vi "Baud Rate Detect.vi"() -> ()   [LabVIEW 2011]
doc: "ID=0x6009"
uses:
  VIs/g_data.ctl
  data/ControlCAN.dll
panel:
  out "label2 4":string="CAN中继状态"
  out "label2 3":string="CAN中继状态"
  out "label2 2":string="CAN中继状态"
  out "label2":string="CAN中继状态"
  in  "help":bool
  in  "close":bool
  in  "DevInd":u32(ring) caption="Device index:" items=["0", "1", "2", "3", "4"]
  in  "SAM":u8(ring) caption="Sample:" items=["Sampling 1 time", "Sampling 3 times"]
  in  "SJW":u8(ring)=1 caption="SJW:" items=["1TQ"=1, "2TQ"=2, "3TQ"=3, "4TQ"=4]
  in  "detect_n":bool
  in  "g_e":dbl=1000.0 caption="To" min=10.0 max=1000.0 step=0.001
  in  "g_b":dbl=10.0 caption="From" min=10.0 max=1000.0 step=0.001
  in  "VCI_CAN_STATUS":T1
  out "Success":bool
  in  "stop":bool
  in  "apply":bool
  in  "detect":bool
  in  "list":i32(listbox)
  in  "Run":bool
  in  "Channel":u32(ring) caption="Channel:" items=["Ch1", "Ch2"]
  in  "DevType":u32(ring)=3 caption="Device type:" items=["USB-CAN"=3, "USB-CAN 2.0"=4]
  # "Kbps"
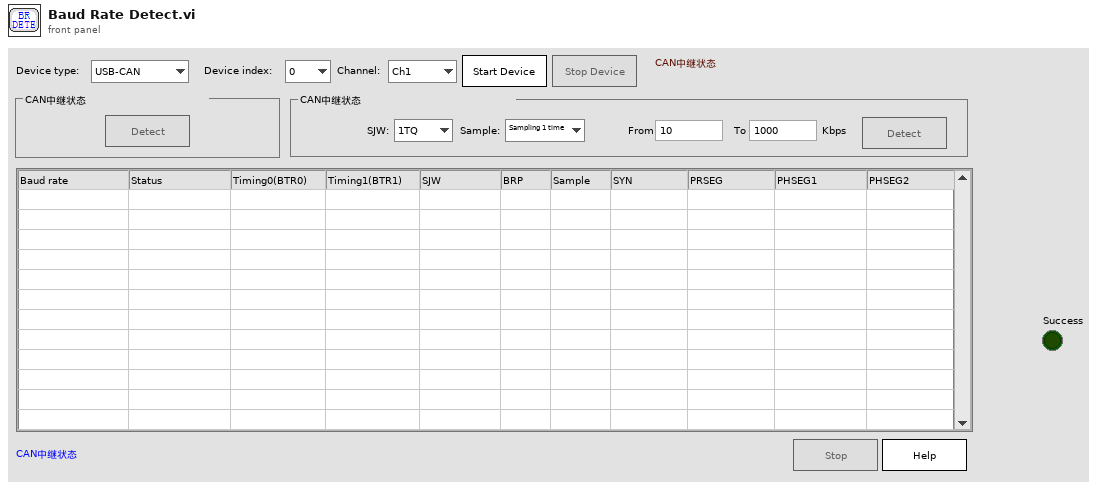
[diagram p1: front panel]
types:
  T1 = cluster{"ErrInterrupt":u8, "regMode":u8, "regStatus":u8, "regALCapture":u8, "regECCapture":u8, "regEWLimit":u8, "regRECounter":u8, "regTECounter":u8, "Reserved":u32}
  T2 = typedef "Baud rate Self Define.ctl" = cluster{"BAUD":u32, "SJW":u8, "BRP":u8, "SAM":u8, "PHS2_SEL":u8, "SYN(nouse)":u8, "PRSEG":u8, "PHSEG1":u8, "PHSEG2":u8}
  T3 = cluster{"AccCode":u32, "AccMask":u32, "Reserved":u32, "Filter":u8, "Timing0":u8, "Timing1":u8, "Mode":u8}
  T4 = typedef "g_data.ctl" = cluster{"b":dbl, "e":dbl}
  T5 = enum8{"Enabled", "Disabled", "Disabled and Grayed Out"}
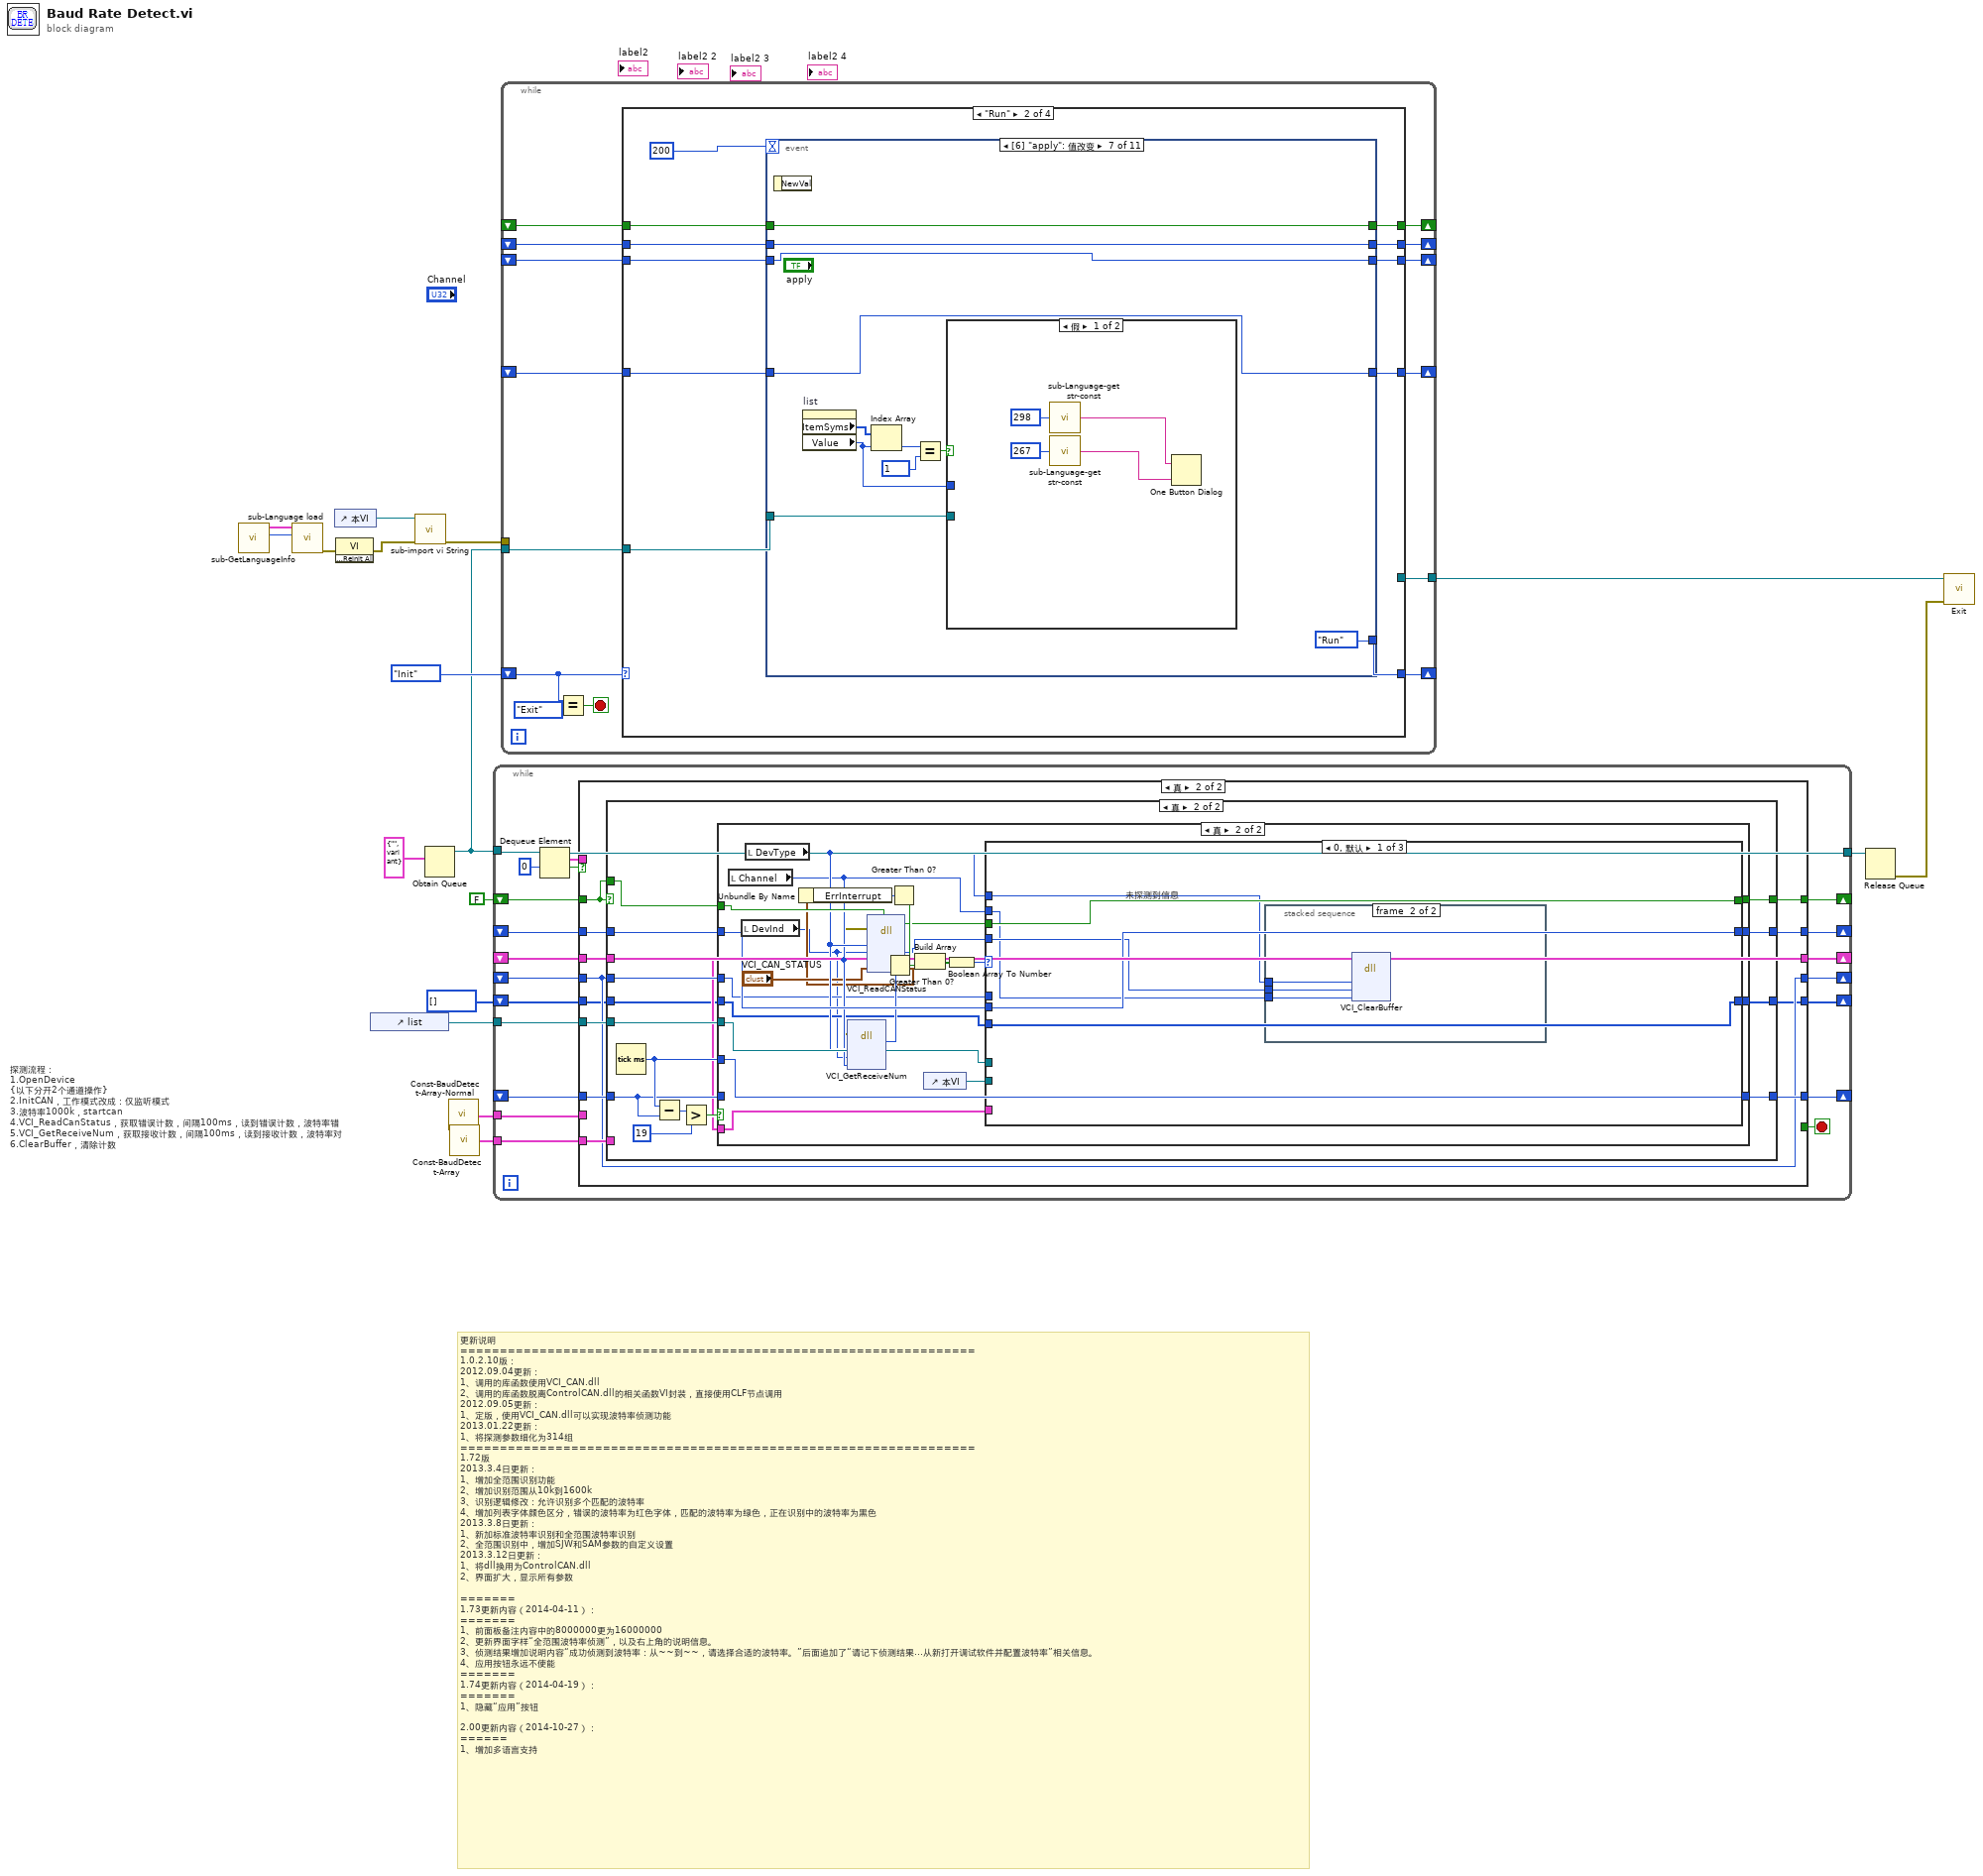
[diagram p0: block diagram]
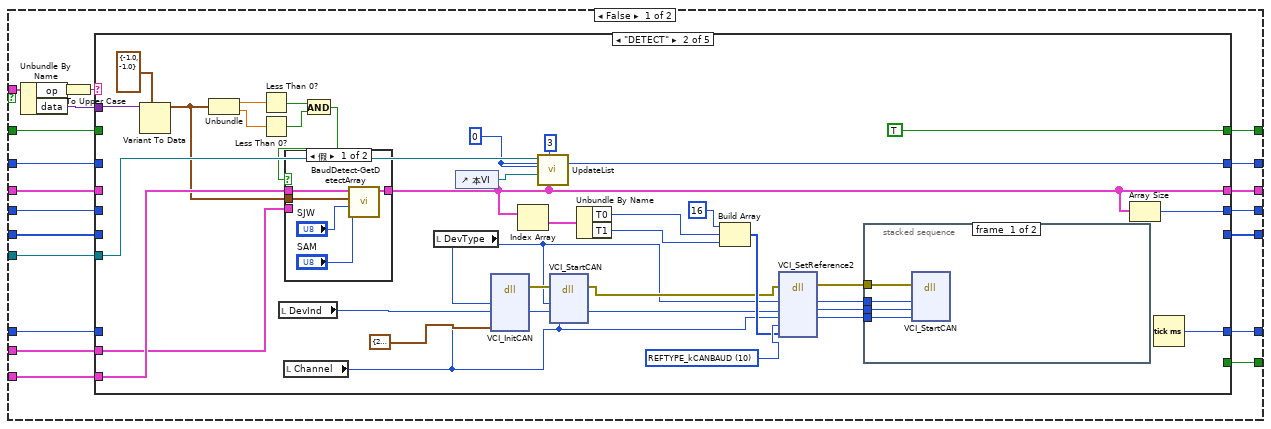
[diagram p2: hidden frame]
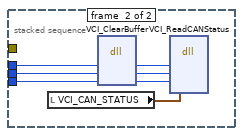
[diagram p4: hidden frame]
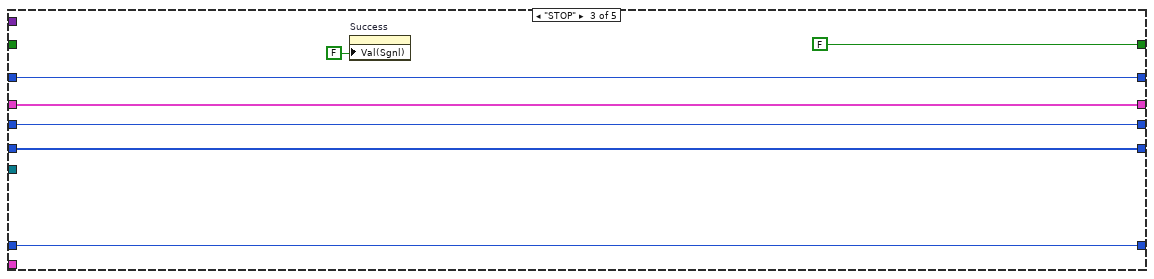
[diagram p6: hidden frame]
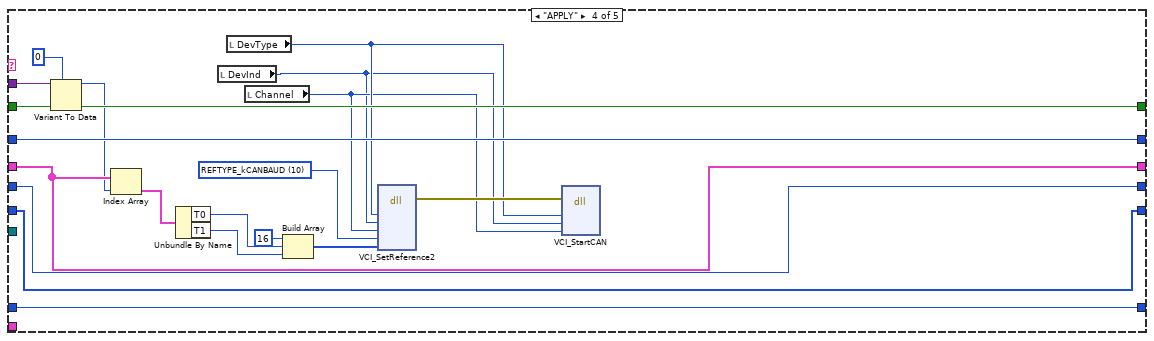
[diagram p7: hidden frame]
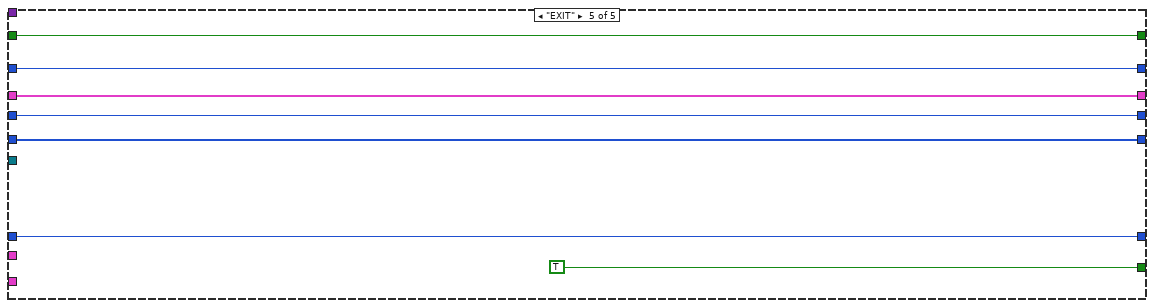
[diagram p8: hidden frame]
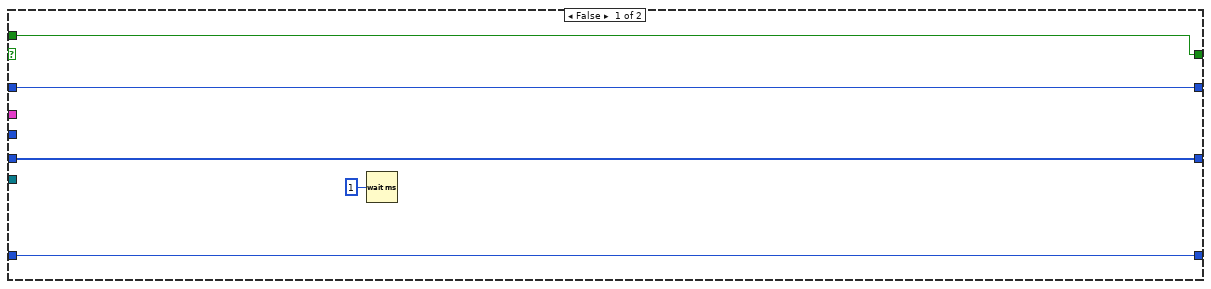
[diagram p9: hidden frame]
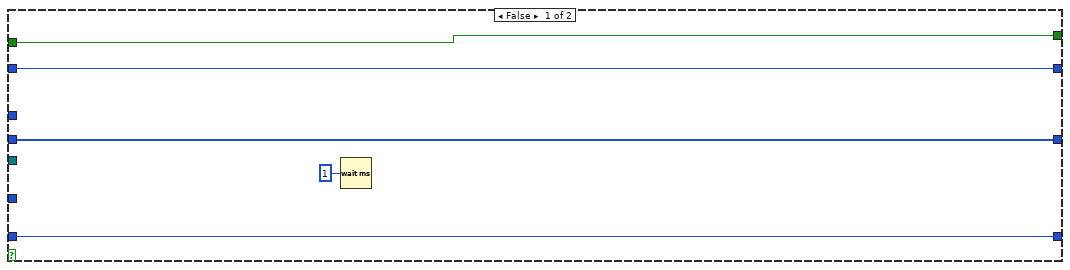
[diagram p10: hidden frame]
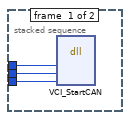
[diagram p11: hidden frame]
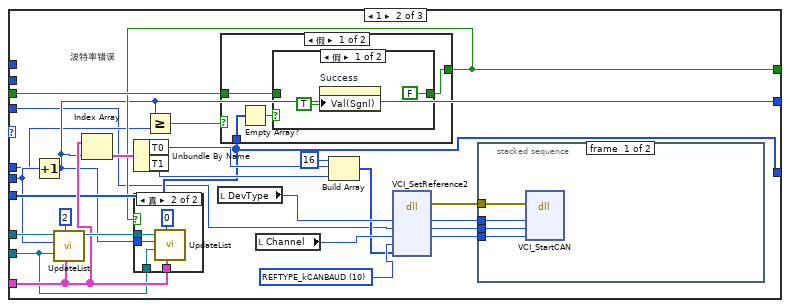
[diagram p12: hidden frame]
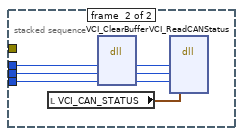
[diagram p14: hidden frame]
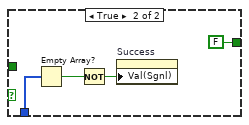
[diagram p16: hidden frame]
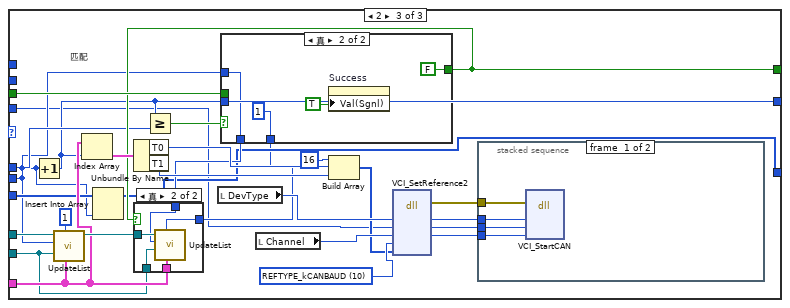
[diagram p17: hidden frame]
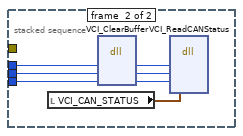
[diagram p19: hidden frame]
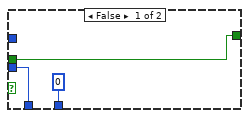
[diagram p20: hidden frame]
diagram:
  # "更新说明\n=================================================================\n1.0.2.10版：\n2012.09.04更新：\n1、调用的库函数使用VCI_CAN.dll\n2、调用的库函数脱离ControlCAN.dll的相关函数VI封装，直接使用CLF节点调用\n2012.09.05更新：\n1、定版，使用VCI_CAN.dll可以实现波特率侦测功能\n2013.01.22更新：\n1、将探测参数细化为314组\n=================================================================\n1.72版\n2013.3.4日更新：\n1、增加全范围识别功能\n2、增加识别范围从10k到1600k\n3、识别逻辑修改：允许识别多个匹配的波特率\n4、增加列表字体颜色区分，错误的波特率为红色字体，匹配的波特率为绿色，正在识别中的波特率为黑色\n2013.3.8日更新：\n1、新加标准波特率识别和全范围波特率识别\n2、全范围识别中，增加SJW和SAM参数的自定义设置\n2013.3.12日更新：\n1、将dll换用为ControlCAN.dll\n2、界面扩大，显示所有参数\n\n=======\n1.73更新内容（2014-04-11）：\n=======\n1、前面板备注内容中的8000000更为16000000\n2、更新界面字样“全范围波特率侦测”，以及右上角的说明信息。\n3、侦测结果增加说明内容“成功侦测到波特率：从~~到~~，请选择合适的波特率。”后面追加了“请记下侦测结果...从新打开调试软件并配置波特率”相关信息。\n4、应用按钮永远不使能\n=======\n1.74更新内容（2014-04-19）：\n=======\n1、隐藏“应用”按钮\n\n2.00更新内容（2014-10-27）：\n======\n1、增加多语言支持"
  # "探测流程：\n1.OpenDevice\n{以下分开2个通道操作}\n2.InitCAN，工作模式改成：仅监听模式\n3.波特率1000k，startcan\n4.VCI_ReadCanStatus，获取错误计数，间隔100ms，读到错误计数，波特率错\n5.VCI_GetReceiveNum，获取接收计数，间隔100ms，读到接收计数，波特率对\n6.ClearBuffer，清除计数"
  n1 = call "sub-GetLanguageInfo.vi"() -> ("selected"=w1:i32, "languages"=w5:cluster{string, "appended path":path, string}[])  [unwired: 10 in]
  n2 = call "sub-Language load.vi"("selected"=w1, "languages"=w5) -> ("error out"=w2:errorcluster)  [unwired: 9 in]
  n3 = control-ref of="本VI"() -> (w6:refnum<vi>)
  n4 = invoke class="VI" method="Default Vals.Reinit All"(error in=w2) -> (error out=w3:errorcluster)  [unwired: 2 in, 2 out]
  n5 = control-ref of="list"() -> (w13:refnum<vi>)
  n6 = call "sub-import vi String.vi"("error in (no error)"=w3, "vi ref"=w6) -> ("error out"=w4:errorcluster)  [unwired: 9 in]
  n7 = Obtain Queue(element data type=cluster{"op":string, "data":variant} {"op"="", "data"=variant}) -> (queue out=w16:refnum<queue>)  [unwired: 4 in, 2 out]
  n8 = call "Const-BaudDetect-Array-Normal.vi"() -> ("DetectArray Nml"=w7:cluster{"T0":u8, "T1":u8, "br_selfdef":T2}[])
  n9 = call "Const-BaudDetect-Array.vi"() -> ("DetectArray"=w10:cluster{"T0":u8, "T1":u8, "br_selfdef":T2}[])
  n10 = while {
    tunnel: w16 -> [w34]
    tunnel: [w33] -> w15
    shift-right: [w31] -> _
    shift-left: FALSE -> [w32]
    shift-right: [w29] -> _
    shift-left: _ -> [w30]
    shift-right: [w28] -> _
    shift-left: _ -> [w27]
    tunnel: w13 -> [w26]
    tunnel: w10 -> [w25]
    shift-right: [w23] -> _
    shift-left: _ -> [w22]
    shift-right: [w21] -> _
    shift-left: _ -> [w24]
    shift-right: [w19] -> _
    shift-left: i32[] [] -> [w20]
    tunnel: w7 -> [w18]
    stop <- w35 stop-if-true
    n11 = Dequeue Element(queue=w34, timeout in ms (-1)=0 ("超时毫秒(-1)")) -> (queue out=w33:refnum<queue>, element=w36:cluster{"op":string, "data":variant}, timed out?=w37:bool)  [unwired: 1 in, 1 out]
    n12 = case shown="真" w37 {
      tunnel: w36 -> [w58 _]
      tunnel: [w56 _] -> w35
      tunnel: w32 -> [w55 w157]
      tunnel: [w54 w156] -> w31
      tunnel: w30 -> [w53 w160]
      tunnel: [w52 w159] -> w29
      tunnel: [w51 w161] -> w28
      tunnel: w27 -> [w50 w162]
      tunnel: w26 -> [w49 w158]
      tunnel: w25 -> [w48 w155]
      tunnel: w24 -> [w47 w153]
      tunnel: [w44 w154] -> w23
      tunnel: w22 -> [w43 w154]
      tunnel: [w42 w153] -> w21
      tunnel: w20 -> [w41 w152]
      tunnel: [w40 w151] -> w19
      tunnel: w18 -> [w39 _]
      frame False {
        n13 = Unbundle By Name(w58) -> ("op"=w46:string, "data"=w45:variant)
        n14 = To Upper Case(1:w46) -> (0:w57:string)
        n15 = case shown="\"DETECT\"" w57 {
          tunnel: [_ _ _ _ TRUE] -> w56
          tunnel: w55 -> [w64 _ _ w143 w149]
          tunnel: [w64 TRUE FALSE w143 w149] -> w54
          tunnel: w53 -> [w63 _ w124 w141 w148]
          tunnel: [w63 w95 w124 w141 w148] -> w52
          tunnel: [w62 w99 w123 w142 w147] -> w51
          tunnel: w50 -> [w62 _ w123 w142 w147]
          tunnel: w49 -> [_ w98 _ _ _]
          tunnel: w48 -> [_ w92 _ _ _]
          tunnel: w47 -> [w60 _ w119 w135 w145]
          tunnel: w45 -> [_ w94 _ w133 _]
          tunnel: [w61 w74 w120 w131 w146] -> w44
          tunnel: w43 -> [w61 _ w120 w131 w146]
          tunnel: [w60 w91 w119 w135 w145] -> w42
          tunnel: w41 -> [w59 _ w118 w134 w144]
          tunnel: [w59 _ w118 w134 w144] -> w40
          tunnel: w39 -> [_ w83 _ _ _]
          frame "假", Default {
          }
          frame "DETECT" {
            w82 = u32 10 items=["REFTYPE_MODE"=0, "REFTYPE_FILTER"=1, "REFTYPE_ACR0"=2, "REFTYPE_AMR0"=6, "REFTYPE_kCANBAUD"=10, "REFTYPE_CANRX_EN"=13, "REFTYPE_UARTBAUD"=14, "REFTYPE_ALL"=15] ("RefType")
            w95 = 0 ("t")
            n16 = Variant To Data(type=T4 {"b"=-1.0, "e"=-1.0} ("g_data"), Variant=w94) -> (data=w89:T4)  [unwired: 1 in, 1 out]
            n17 = Unbundle(w89) -> ("b"=w88:dbl, "e"=w87:dbl)
            n18 = Less Than 0?(x=w88) -> (x < 0?=w86:bool)
            n19 = Less Than 0?(x=w87) -> (x < 0?=w85:bool)
            n20 = local read "DevInd"() -> (w66:u32)
            n21 = local read "Channel"() -> (w65:u32)
            n22 = And(x=w86, y=w85) -> (x .and. y?=w84:bool)
            n23 = case shown="假" w84 {
              tunnel: w92 -> [w116 _]
              tunnel: [w115 w117] -> w74
              tunnel: w89 -> [w114 _]
              tunnel: w83 -> [_ w117]
              frame False {
                n24 = call "BaudDetect-GetDetectArray.vi"("SAM"="SAM", "SJW"="SJW", "g_data"=w114, "DetectArray in"=w116) -> ("DetectArray out"=w115:cluster{"T0":u8, "T1":u8, "br_selfdef":T2}[])  [unwired: 7 in]
              }
              frame True {
              }
            }
            n25 = local read "DevType"() -> (w67:u32)
            n26 = control-ref of="本VI"() -> (w90:refnum<vi>)
            n27 = dll-call lib="PTH1[abs ZHost_E工作Tnewcodewith eng verUSB CAN Tool2.02dataControlCAN.dll" fn="VCI_InitCAN"("DeviceType"=w67, "DeviceInd"=w66, "CANInd"=w65, "pInitConfig"=T3 {"AccCode"=2147483648, "AccMask"=4294967295, "Reserved"=0, "Filter"=1, "Timing0"=0, "Timing1"=20, "Mode"=1}) -> (error out=w96:errorcluster, "DeviceInd"=w70:u32)  [unwired: 7 in, 1 out]
            n28 = Index Array(array=w74) -> (element=w73:cluster{"T0":u8, "T1":u8, "br_selfdef":T2})  [unwired: 1 in]
            n29 = call "UpdateList.vi"("DetectArray"=w74, "Operation"=u8 3, "VI引用句柄"=w90, "Baud Rate"=w95, "list"=w98) -> ()  [unwired: 6 in, 1 out]
            n30 = dll-call lib="PTH1[abs ZHost_E工作Tnewcodewith eng verUSB CAN Tool2.02dataControlCAN.dll" fn="VCI_StartCAN"(error in=w96, "DeviceType"=w67, "DeciceInd"=w70, "CANInd"=w65) -> (error out=w76:errorcluster, "DeciceInd"=w69:u32)  [unwired: 5 in, 1 out]
            n31 = Unbundle By Name(w73) -> ("T0"=w72:u8, "T1"=w71:u8)
            n32 = Build Array(u8 16 ("元素"), w72, w71) -> (w77:u8[])
            n33 = dll-call lib="PTH1[abs ZHost_E工作Tnewcodewith eng verUSB CAN Tool2.02dataControlCAN.dll" fn="VCI_SetReference2" label="VCI_SetReference"(error in=w76, "DeviceType"=w67, "DeviceInd"=w69, "CANInd"=w65, "RefType"=w82, "pData"=w77) -> (error out=w81:errorcluster, "DeviceType"=w80:u32, "DeviceInd"=w79:u32, "CANInd"=w78:u32)  [unwired: 5 in, 1 out]
            n34 = stacked-sequence {
              tunnel: w81 -> [w104 _]
              tunnel: w80 -> [w103 w107]
              tunnel: w79 -> [w102 w106]
              tunnel: w78 -> [w101 w105]
              frame #0 {
                n35 = dll-call lib="PTH1[abs ZHost_E工作Tnewcodewith eng verUSB CAN Tool2.02dataControlCAN.dll" fn="VCI_StartCAN"(error in=w104, "DeviceType"=w103, "DeciceInd"=w102, "CANInd"=w101) -> ()  [unwired: 6 in, 2 out]
              }
              frame #1 {
                n36 = local read "VCI_CAN_STATUS"() -> (w108:T1)
                n37 = dll-call lib="PTH1[abs ZHost_E工作Tnewcodewith eng verUSB CAN Tool2.02dataControlCAN.dll" fn="VCI_ClearBuffer"("DeviceType"=w107, "DeciceInd"=w106, "CANInd"=w105) -> ("DeviceType"=w111:u32, "DeciceInd"=w110:u32, "CANInd"=w109:u32)  [unwired: 4 in, 2 out]
                n38 = dll-call lib="PTH1[abs ZHost_E工作Tnewcodewith eng verUSB CAN Tool2.02dataControlCAN.dll" fn="VCI_ReadCANStatus"("DeviceType"=w111, "DeciceInd"=w110, "CANInd"=w109, "pCANStatus"=w108) -> ()  [unwired: 8 in, 2 out]
              }
            }
            n39 = Array Size(array=w74) -> (size(s)=w91:i32)
            n40 = Tick Count (ms)() -> (millisecond timer value=w99:u32)
          }
          frame "STOP" {
            n41 = property on="Success" class="Bool (严格)"("Val(Sgnl)"=FALSE ("值(信号)")) -> ()  [unwired: 2 in, 2 out]
          }
          frame "APPLY" {
            w140 = u32 10 items=["REFTYPE_MODE"=0, "REFTYPE_FILTER"=1, "REFTYPE_ACR0"=2, "REFTYPE_AMR0"=6, "REFTYPE_kCANBAUD"=10, "REFTYPE_CANRX_EN"=13, "REFTYPE_UARTBAUD"=14, "REFTYPE_ALL"=15] ("RefType")
            n42 = Variant To Data(type=0 ("list"), Variant=w133) -> (data=w127:i32)  [unwired: 1 in, 1 out]
            n43 = Index Array(array=w131, index=w127) -> (element=w130:cluster{"T0":u8, "T1":u8, "br_selfdef":T2})
            n44 = Unbundle By Name(w130) -> ("T0"=w129:u8, "T1"=w128:u8)
            n45 = local read "DevInd"() -> (w125:u32)
            n46 = local read "DevType"() -> (w137:u32)
            n47 = local read "Channel"() -> (w136:u32)
            n48 = Build Array(u8 16 ("元素"), w129, w128) -> (w139:u8[])
            n49 = dll-call lib="PTH1[abs ZHost_E工作Tnewcodewith eng verUSB CAN Tool2.02dataControlCAN.dll" fn="VCI_SetReference2" label="VCI_SetReference"("DeviceType"=w137, "DeviceInd"=w125, "CANInd"=w136, "RefType"=w140, "pData"=w139) -> (error out=w138:errorcluster)  [unwired: 9 in, 1 out]
            n50 = dll-call lib="PTH1[abs ZHost_E工作Tnewcodewith eng verUSB CAN Tool2.02dataControlCAN.dll" fn="VCI_StartCAN"(error in=w138, "DeviceType"=w137, "DeciceInd"=w125, "CANInd"=w136) -> ()  [unwired: 6 in, 2 out]
          }
          frame "EXIT" {
          }
        }
      }
      frame True {
        n51 = case shown="真" w157 {
          tunnel: w162 -> [w167 w178]
          tunnel: [w167 w177] -> w161
          tunnel: w160 -> [w166 w176]
          tunnel: [w166 w175] -> w159
          tunnel: w158 -> [_ w174]
          tunnel: w157 -> [w165 w173]
          tunnel: [w165 w172] -> w156
          tunnel: w155 -> [_ _]
          tunnel: w153 -> [_ w171]
          tunnel: w154 -> [_ w170]
          tunnel: w152 -> [w163 w169]
          tunnel: [w163 w168] -> w151
          frame False {
            n52 = Wait (ms)(milliseconds to wait=u32 1 ("等待时间（毫秒）")) -> ()  [unwired: 1 out]
          }
          frame True {
            n53 = Tick Count (ms)() -> (millisecond timer value=w179:u32)
            n54 = Subtract(x=w179, y=w178) -> (x-y=w182:u32)
            n55 = Greater?(x=w182, y=u32 19) -> (0:w180:bool)
            n56 = case shown="真" w180 {
              tunnel: w179 -> [_ w211]
              tunnel: w178 -> [w187 _]
              tunnel: [w187 w211] -> w177
              tunnel: w176 -> [w186 w207]
              tunnel: [w186 w206] -> w175
              tunnel: w174 -> [_ w205]
              tunnel: w173 -> [w185 w204]
              tunnel: [w185 w203] -> w172
              tunnel: w170 -> [_ w201]
              tunnel: w171 -> [_ w194]
              tunnel: w169 -> [w183 w193]
              tunnel: [w183 w192] -> w168
              frame False {
                n57 = Wait (ms)(milliseconds to wait=u32 1 ("等待时间（毫秒）")) -> ()  [unwired: 1 out]
              }
              frame True {
                n58 = local read "Channel"() -> (w199:u32)
                n59 = local read "DevInd"() -> (w189:u32)
                n60 = local read "DevType"() -> (w200:u32)
                n61 = dll-call lib="PTH1[abs ZHost_E工作Tnewcodewith eng verUSB CAN Tool2.02dataControlCAN.dll" fn="VCI_ReadCANStatus"("DeviceType"=w200, "DeciceInd"=w189, "CANInd"=w199, "pCANStatus"="VCI_CAN_STATUS") -> (error out=w195:errorcluster, "DeciceInd"=w188:u32, "pCANStatus"=w196:T1)  [unwired: 6 in, 1 out]
                n62 = Unbundle By Name(w196) -> ("ErrInterrupt"=w202:u8)
                n63 = dll-call lib="PTH1[abs ZHost_E工作Tnewcodewith eng verUSB CAN Tool2.02dataControlCAN.dll" fn="VCI_GetReceiveNum"(error in=w195, "DeviceType"=w200, "DeciceInd"=w189, "CANInd"=w199) -> ("返回类型"=w198:u32)  [unwired: 5 in, 2 out]
                n64 = Greater Than 0?(x=w198) -> (x > 0?=w209:bool)
                n65 = Greater Than 0?(x=w202) -> (x > 0?=w210:bool)
                n66 = Build Array(w210, w209) -> (w208:bool[])
                n67 = control-ref of="本VI"() -> (w191:refnum<vi>)
                n68 = Boolean Array To Number(Boolean array=w208) -> (number=w190:u32)
                n69 = case shown="0, 默认" w190 {
                  tunnel: w207 -> [w217 w227 w279]
                  tunnel: [w217 w226 w278] -> w206
                  tunnel: w200 -> [w214 _ _]
                  tunnel: w199 -> [w212 _ _]
                  tunnel: w205 -> [_ w248 w303]
                  tunnel: w204 -> [w216 w244 w299]
                  tunnel: [w216 w229 w284] -> w203
                  tunnel: w201 -> [_ w235 w290]
                  tunnel: w194 -> [_ w225 w280]
                  tunnel: w193 -> [w215 w231 w286]
                  tunnel: [w215 w231 w281] -> w192
                  tunnel: w191 -> [_ w228 w283]
                  tunnel: w188 -> [w213 w224 w276]
                  frame 0, Default {
                    # "未探测到信息"
                    n70 = stacked-sequence {
                      tunnel: w214 -> [w220 w223]
                      tunnel: w213 -> [w219 w222]
                      tunnel: w212 -> [w218 w221]
                      frame #0 {
                        n71 = dll-call lib="PTH1[abs ZHost_E工作Tnewcodewith eng verUSB CAN Tool2.02dataControlCAN.dll" fn="VCI_StartCAN"("DeviceType"=w220, "DeciceInd"=w219, "CANInd"=w218) -> ()  [unwired: 7 in, 2 out]
                      }
                      frame #1 {
                        n72 = dll-call lib="PTH1[abs ZHost_E工作Tnewcodewith eng verUSB CAN Tool2.02dataControlCAN.dll" fn="VCI_ClearBuffer"("DeviceType"=w223, "DeciceInd"=w222, "CANInd"=w221) -> ()  [unwired: 7 in, 2 out]
                      }
                    }
                  }
                  frame 1 {
                    w241 = u32 10 items=["REFTYPE_MODE"=0, "REFTYPE_FILTER"=1, "REFTYPE_ACR0"=2, "REFTYPE_AMR0"=6, "REFTYPE_kCANBAUD"=10, "REFTYPE_CANRX_EN"=13, "REFTYPE_UARTBAUD"=14, "REFTYPE_ALL"=15] ("RefType")
                    # "波特率错误"
                    n73 = Increment(x=w227) -> (x+1=w226:i32)
                    n74 = call "UpdateList.vi"("DetectArray"=w235, "Operation"=u8 2, "VI引用句柄"=w228, "Baud Rate"=w227, "list"=w248) -> ("list out"=w246:refnum<vi>)  [unwired: 6 in]
                    n75 = Index Array(array=w235, index=w226) -> (element=w234:cluster{"T0":u8, "T1":u8, "br_selfdef":T2})
                    n76 = Unbundle By Name(w234) -> ("T0"=w232:u8, "T1"=w233:u8)
                    n77 = Greater Or Equal?(x=w226, y=w225) -> (x >= y?=w245:bool)
                    n78 = local read "DevType"() -> (w243:u32)
                    n79 = case shown="假" w245 {
                      tunnel: w244 -> [w266 _]
                      tunnel: [w265 FALSE] -> w229
                      tunnel: w231 -> [w268 w274]
                      frame False {
                        n80 = Empty Array?(array=w268) -> (empty?=w267:bool)
                        n81 = case shown="假" w267 {
                          tunnel: w266 -> [_ w271]
                          tunnel: [FALSE w271] -> w265
                          frame False {
                            n82 = property on="Success" class="Bool (严格)"("Val(Sgnl)"=TRUE ("值(信号)")) -> ()  [unwired: 2 in, 2 out]
                          }
                          frame True {
                          }
                        }
                      }
                      frame True {
                        n83 = Empty Array?(array=w274) -> (empty?=w273:bool)
                        n84 = Not(x=w273) -> (.not. x?=w272:bool)
                        n85 = property on="Success" class="Bool (严格)"("Val(Sgnl)"=w272) -> ()  [unwired: 2 in, 2 out]
                      }
                    }
                    n86 = case shown="真" w229 {
                      tunnel: w246 -> [_ w253]
                      tunnel: w226 -> [_ w251]
                      tunnel: w235 -> [_ w250]
                      tunnel: w228 -> [_ w249]
                      frame False {
                      }
                      frame True {
                        n87 = call "UpdateList.vi"("DetectArray"=w250, "Operation"=u8 0, "VI引用句柄"=w249, "Baud Rate"=w251, "list"=w253) -> ()  [unwired: 6 in, 1 out]
                      }
                    }
                    n88 = local read "Channel"() -> (w242:u32)
                    n89 = Build Array(u8 16 ("元素"), w232, w233) -> (w240:u8[])
                    n90 = dll-call lib="PTH1[abs ZHost_E工作Tnewcodewith eng verUSB CAN Tool2.02dataControlCAN.dll" fn="VCI_SetReference2" label="VCI_SetReference"("DeviceType"=w243, "DeviceInd"=w224, "CANInd"=w242, "RefType"=w241, "pData"=w240) -> (error out=w239:errorcluster, "DeviceType"=w238:u32, "DeviceInd"=w237:u32, "CANInd"=w236:u32)  [unwired: 6 in, 1 out]
                    n91 = stacked-sequence {
                      tunnel: w239 -> [w257 _]
                      tunnel: w238 -> [w256 w260]
                      tunnel: w237 -> [w255 w259]
                      tunnel: w236 -> [w254 w258]
                      frame #0 {
                        n92 = dll-call lib="PTH1[abs ZHost_E工作Tnewcodewith eng verUSB CAN Tool2.02dataControlCAN.dll" fn="VCI_StartCAN"(error in=w257, "DeviceType"=w256, "DeciceInd"=w255, "CANInd"=w254) -> ()  [unwired: 6 in, 2 out]
                      }
                      frame #1 {
                        n93 = local read "VCI_CAN_STATUS"() -> (w261:T1)
                        n94 = dll-call lib="PTH1[abs ZHost_E工作Tnewcodewith eng verUSB CAN Tool2.02dataControlCAN.dll" fn="VCI_ClearBuffer"("DeviceType"=w260, "DeciceInd"=w259, "CANInd"=w258) -> ("DeviceType"=w264:u32, "DeciceInd"=w263:u32, "CANInd"=w262:u32)  [unwired: 4 in, 2 out]
                        n95 = dll-call lib="PTH1[abs ZHost_E工作Tnewcodewith eng verUSB CAN Tool2.02dataControlCAN.dll" fn="VCI_ReadCANStatus"("DeviceType"=w264, "DeciceInd"=w263, "CANInd"=w262, "pCANStatus"=w261) -> ()  [unwired: 8 in, 2 out]
                      }
                    }
                  }
                  frame 2 {
                    w296 = u32 10 items=["REFTYPE_MODE"=0, "REFTYPE_FILTER"=1, "REFTYPE_ACR0"=2, "REFTYPE_AMR0"=6, "REFTYPE_kCANBAUD"=10, "REFTYPE_CANRX_EN"=13, "REFTYPE_UARTBAUD"=14, "REFTYPE_ALL"=15] ("RefType")
                    # "匹配"
                    n96 = Increment(x=w279) -> (x+1=w278:i32)
                    n97 = call "UpdateList.vi"("DetectArray"=w290, "Operation"=u8 1, "VI引用句柄"=w283, "Baud Rate"=w279, "list"=w303) -> ("list out"=w301:refnum<vi>)  [unwired: 6 in]
                    n98 = Index Array(array=w290, index=w278) -> (element=w289:cluster{"T0":u8, "T1":u8, "br_selfdef":T2})
                    n99 = Insert Into Array(array=w286, new element=w279) -> (w281:i32[])  [unwired: 1 in]
                    n100 = Unbundle By Name(w289) -> ("T0"=w287:u8, "T1"=w288:u8)
                    n101 = Greater Or Equal?(x=w278, y=w280) -> (x >= y?=w300:bool)
                    n102 = local read "DevType"() -> (w298:u32)
                    n103 = case shown="真" w300 {
                      tunnel: w299 -> [w322 _]
                      tunnel: [w322 FALSE] -> w284
                      tunnel: [u8 0 ("Operation") u8 1 ("Operation")] -> w277
                      tunnel: w279 -> [_ w323]
                      tunnel: [w320 w323] -> w282
                      tunnel: w278 -> [w320 _]
                      frame False {
                      }
                      frame True {
                        n104 = property on="Success" class="Bool (严格)"("Val(Sgnl)"=TRUE ("值(信号)")) -> ()  [unwired: 2 in, 2 out]
                      }
                    }
                    n105 = case shown="真" w284 {
                      tunnel: w301 -> [_ w308]
                      tunnel: w290 -> [_ w307]
                      tunnel: w283 -> [_ w306]
                      tunnel: w277 -> [_ w305]
                      tunnel: w282 -> [_ w304]
                      frame False {
                      }
                      frame True {
                        n106 = call "UpdateList.vi"("DetectArray"=w307, "Operation"=w305, "VI引用句柄"=w306, "Baud Rate"=w304, "list"=w308) -> ()  [unwired: 6 in, 1 out]
                      }
                    }
                    n107 = local read "Channel"() -> (w297:u32)
                    n108 = Build Array(u8 16 ("元素"), w287, w288) -> (w295:u8[])
                    n109 = dll-call lib="PTH1[abs ZHost_E工作Tnewcodewith eng verUSB CAN Tool2.02dataControlCAN.dll" fn="VCI_SetReference2" label="VCI_SetReference"("DeviceType"=w298, "DeviceInd"=w276, "CANInd"=w297, "RefType"=w296, "pData"=w295) -> (error out=w294:errorcluster, "DeviceType"=w293:u32, "DeviceInd"=w292:u32, "CANInd"=w291:u32)  [unwired: 6 in, 1 out]
                    n110 = stacked-sequence {
                      tunnel: w294 -> [w312 _]
                      tunnel: w293 -> [w311 w315]
                      tunnel: w292 -> [w310 w314]
                      tunnel: w291 -> [w309 w313]
                      frame #0 {
                        n111 = dll-call lib="PTH1[abs ZHost_E工作Tnewcodewith eng verUSB CAN Tool2.02dataControlCAN.dll" fn="VCI_StartCAN"(error in=w312, "DeviceType"=w311, "DeciceInd"=w310, "CANInd"=w309) -> ()  [unwired: 6 in, 2 out]
                      }
                      frame #1 {
                        n112 = local read "VCI_CAN_STATUS"() -> (w316:T1)
                        n113 = dll-call lib="PTH1[abs ZHost_E工作Tnewcodewith eng verUSB CAN Tool2.02dataControlCAN.dll" fn="VCI_ClearBuffer"("DeviceType"=w315, "DeciceInd"=w314, "CANInd"=w313) -> ("DeviceType"=w319:u32, "DeciceInd"=w318:u32, "CANInd"=w317:u32)  [unwired: 4 in, 2 out]
                        n114 = dll-call lib="PTH1[abs ZHost_E工作Tnewcodewith eng verUSB CAN Tool2.02dataControlCAN.dll" fn="VCI_ReadCANStatus"("DeviceType"=w319, "DeciceInd"=w318, "CANInd"=w317, "pCANStatus"=w316) -> ()  [unwired: 8 in, 2 out]
                      }
                    }
                  }
                }
              }
            }
          }
        }
      }
    }
  }
  n115 = while {
    shift-right: [w337] -> _
    shift-left: enum16{"Init", "Run", "Release", "Exit"}."Init" -> [w338]
    shift-right: [w336] -> _
    shift-left: _ -> [w335]
    tunnel: w16 -> [w334]
    tunnel: [w333] -> w11
    shift-right: [w331] -> _
    shift-left: _ -> [w332]
    shift-right: [w328] -> _
    shift-left: _ -> [w330]
    shift-right: [w327] -> _
    shift-left: _ -> [w329]
    tunnel: w4 -> [_]
    stop <- w339 stop-if-true
    n116 = Equal?(x=w338, y=enum16{"Init", "Run", "Release", "Exit"}."Exit") -> (x = y?=w339:bool)
    n117 = case shown="\"Run\"" w338 {
      tunnel: [enum16{"Init", "Run", "Release", "Exit"}."Run" w358 enum16{"Init", "Run", "Release", "Exit"}."Exit" enum16{"Init", "Run", "Release", "Exit"}."Exit"] -> w337
      tunnel: [_ w357 _ _] -> w336
      tunnel: w335 -> [_ w356 w505 _]
      tunnel: w334 -> [_ w355 w504 _]
      tunnel: [_ _ _ w509] -> w333
      tunnel: w332 -> [_ w354 _ _]
      tunnel: [-1 w353 _ _] -> w331
      tunnel: w330 -> [_ w351 _ _]
      tunnel: w329 -> [_ w350 _ _]
      tunnel: [_ w349 _ _] -> w328
      tunnel: [u32 255 ("DevInd") w348 _ _] -> w327
      frame "Init", Default {
        w344 = T5."Enabled" ("禁用")
        w345 = T5."Disabled and Grayed Out" ("禁用")
        n118 = property on="list" class="MCListbox (严格)"("ItemNames"=string[][] [] ("项名")) -> ()  [unwired: 2 in, 2 out]
        n119 = property on="list" class="MCListbox (严格)"("Value"=-1 ("list")) -> ()  [unwired: 2 in, 2 out]
        n120 = property on="Channel" class="Ring (严格)"("DisabledEnum"=w344) -> ()  [unwired: 2 in, 2 out]
        n121 = property on="DevType" class="Ring (严格)"("DisabledEnum"=w344) -> ()  [unwired: 2 in, 2 out]
        n122 = property on="apply" class="Bool"("DisabledEnum"=w345) -> ()  [unwired: 2 in, 2 out]
        n123 = property on="stop" class="Bool"("DisabledEnum"=w345) -> ()  [unwired: 2 in, 2 out]
        n124 = property on="detect" class="Bool"("DisabledEnum"=w345) -> ()  [unwired: 2 in, 2 out]
      }
      frame "Run" {
        n125 = event shown="[6] \"apply\": 值改变" {
          selector: _ -> [_ _ _ _ _ _ _ _ _ _ _]
          dyn-events: _ -> [_ _ _ _ _ _ _ _ _ _ _]
          timeout: 200 -> [_ _ _ _ _ _ _ _ _ _ _]
          tunnel: [enum16{"Init", "Run", "Release", "Exit"}."Run" enum16{"Init", "Run", "Release", "Exit"}."Release" enum16{"Init", "Run", "Release", "Exit"}."Run" enum16{"Init", "Run", "Release", "Exit"}."Run" enum16{"Init", "Run", "Release", "Exit"}."Run" enum16{"Init", "Run", "Release", "Exit"}."Run" enum16{"Init", "Run", "Release", "Exit"}."Run" enum16{"Init", "Run", "Release", "Exit"}."Run" enum16{"Init", "Run", "Release", "Exit"}."Run" enum16{"Init", "Run", "Release", "Exit"}."Run" enum16{"Init", "Run", "Release", "Exit"}."Run"] -> w358
          tunnel: [w362 w369 w372 w398 w418 w431 w442 w458 w463 w488 w502] -> w357
          tunnel: w356 -> [w362 w369 _ w398 w418 w431 w442 w458 w463 w488 w502]
          tunnel: w355 -> [_ _ _ _ w417 w430 w441 w457 _ _ _]
          tunnel: w354 -> [w361 w367 w377 w397 _ _ w435 _ w462 w484 w501]
          tunnel: [w361 w367 w377 w397 0 1 w435 -1 w462 -1 w501] -> w353
          tunnel: w351 -> [w360 w365 w373 w395 w406 w422 w434 w454 w461 w476 w500]
          tunnel: w350 -> [w359 w364 w374 w392 w405 w421 w433 w453 w460 w475 w499]
          tunnel: [w360 w365 w376 w395 w406 w422 w434 w454 w461 w476 w500] -> w349
          tunnel: [w359 w364 w375 w392 w405 w421 w433 w453 w460 w475 w499] -> w348
          event Timeout {
            n126 = event-data() -> ()  [unwired: 1 in, 1 out]
          }
          event Panel Close? {
            n127 = event-data() -> ()  [unwired: 1 in, 1 out]
            n128 = local read "DevInd"() -> (w366:u32)
            n129 = local read "DevType"() -> (w368:u32)
            n130 = dll-call lib="PTH1[abs ZHost_E工作Tnewcodewith eng verUSB CAN Tool2.02dataControlCAN.dll" fn="VCI_CloseDevice"("DevType"=w368, "DevIndex"=w366) -> ()  [unwired: 6 in, 2 out]
            n131 = event-data("Discard?"=TRUE ("放弃？")) -> ()  [unwired: 1 in, 1 out]
          }
          event "Run": Value Change {
            n132 = event-data() -> ()  [unwired: 1 in, 1 out]
            n133 = stacked-sequence {
              tunnel: [_ w385] -> w372
              tunnel: [_ "DevType"] -> w376
              tunnel: [_ "DevInd"] -> w375
              tunnel: w374 -> [w382 _]
              tunnel: w373 -> [w381 _]
              frame #0 {
                n134 = case shown="99.." w382 {
                  selector: w382 -> [w383 _]
                  tunnel: w381 -> [w384 _]
                  frame 0, Default {
                    n135 = dll-call lib="PTH1[abs ZHost_E工作Tnewcodewith eng verUSB CAN Tool2.02dataControlCAN.dll" fn="VCI_CloseDevice"("DeviceType"=w384, "DeviceInd"=w383) -> ()  [unwired: 6 in, 2 out]
                  }
                  frame 99.. {
                  }
                }
              }
              frame #1 {
                n136 = dll-call lib="PTH1[abs ZHost_E工作Tnewcodewith eng verUSB CAN Tool2.02dataControlCAN.dll" fn="VCI_OpenDevice"("DevType"="DevType", "DevIndex"="DevInd", "Reserved"=u32 0) -> ("返回类型"=w389:u32)  [unwired: 6 in, 2 out]
                n137 = Equal?(x=w389, y=u32 1) -> (x = y?=w385:bool)
              }
            }
            n138 = case shown="真" w372 {
              tunnel: w372 -> [_ _]
              frame False {
              }
              frame True {
                w380 = 0
                w379 = 2
                n139 = property on="close" class="Bool"("DisabledEnum"=w380) -> ()  [unwired: 2 in, 2 out]
                n140 = property on="Run" class="Bool"("DisabledEnum"=w379) -> ()  [unwired: 2 in, 2 out]
                n141 = property on="apply" class="Bool"("DisabledEnum"=w379) -> ()  [unwired: 2 in, 2 out]
                n142 = property on="stop" class="Bool"("DisabledEnum"=w379) -> ()  [unwired: 2 in, 2 out]
                n143 = property on="detect" class="Bool"("DisabledEnum"=w380) -> ()  [unwired: 2 in, 2 out]
                n144 = property on="DevType" class="Ring (严格)"("DisabledEnum"=w379) -> ()  [unwired: 2 in, 2 out]
                n145 = property on="DevInd" class="Ring (严格)"("DisabledEnum"=w379) -> ()  [unwired: 2 in, 2 out]
                n146 = property on="Channel" class="Ring (严格)"("DisabledEnum"=w379) -> ()  [unwired: 2 in, 2 out]
                n147 = property on="detect_n" class="Bool"("DisabledEnum"=w380) -> ()  [unwired: 2 in, 2 out]
              }
            }
          }
          event "close": Value Change {
            n148 = event-data() -> ()  [unwired: 1 in, 1 out]
            n149 = case shown="0, 默认" w392 {
              tunnel: w395 -> [w401 _]
              tunnel: w392 -> [w400 _]
              tunnel: [w399 _] -> w394
              frame 0, Default {
                n150 = dll-call lib="PTH1[abs ZHost_E工作Tnewcodewith eng verUSB CAN Tool2.02dataControlCAN.dll" fn="VCI_CloseDevice"("DeviceType"=w401, "DeviceInd"=w400) -> ("返回类型"=w399:u32)  [unwired: 5 in, 2 out]
              }
              frame 99.. {
              }
            }
            n151 = Equal?(x=u32 1, y=w394) -> (x = y?=w391:bool)
            n152 = case shown="真" w391 {
              frame False {
              }
              frame True {
                w403 = 2
                w402 = 0
                n153 = property on="close" class="Bool"("DisabledEnum"=w403) -> ()  [unwired: 2 in, 2 out]
                n154 = property on="apply" class="Bool"("DisabledEnum"=w403) -> ()  [unwired: 2 in, 2 out]
                n155 = property on="stop" class="Bool"("DisabledEnum"=w403) -> ()  [unwired: 2 in, 2 out]
                n156 = property on="DevType" class="Ring (严格)"("DisabledEnum"=w402) -> ()  [unwired: 2 in, 2 out]
                n157 = property on="DevInd" class="Ring (严格)"("DisabledEnum"=w402) -> ()  [unwired: 2 in, 2 out]
                n158 = property on="detect" class="Bool"("DisabledEnum"=w403) -> ()  [unwired: 2 in, 2 out]
                n159 = property on="Channel" class="Ring (严格)"("DisabledEnum"=w402) -> ()  [unwired: 2 in, 2 out]
                n160 = property on="Run" class="Bool"("DisabledEnum"=w402) -> ()  [unwired: 2 in, 2 out]
                n161 = property on="detect_n" class="Bool"("DisabledEnum"=w403) -> ()  [unwired: 2 in, 2 out]
              }
            }
          }
          event "detect": Value Change {
            w409 = T5."Disabled and Grayed Out" ("禁用")
            w404 = T5."Disabled and Grayed Out" ("禁用")
            n162 = event-data() -> ()  [unwired: 1 in, 1 out]
            n163 = Bundle By Name(cluster=T4 {"b"=-1.0, "e"=-1.0} ("g_data"), "b"="g_b", "e"="g_e") -> (w408:T4)
            n164 = property class="VI"("Front Panel.Closeable"=FALSE ("前面板窗口:可关闭")) -> ()  [unwired: 2 in, 2 out]
            n165 = Bundle By Name(cluster=cluster{"op":string, "data":variant} {"op"="DETECT", "data"=variant}, "data"=w408) -> (w413:cluster{"op":string, "data":variant})
            n166 = property on="close" class="Bool"("DisabledEnum"=w404) -> ()  [unwired: 2 in, 2 out]
            n167 = Enqueue Element(queue=w417, element=w413) -> ()  [unwired: 2 in, 3 out]
            n168 = property on="g_e" class="DigNum (严格)"("DisabledEnum"=w404) -> ()  [unwired: 2 in, 2 out]
            n169 = property on="SAM" class="Ring (严格)"("DisabledEnum"=w404) -> ()  [unwired: 2 in, 2 out]
            n170 = property on="SJW" class="Ring (严格)"("DisabledEnum"=w404) -> ()  [unwired: 2 in, 2 out]
            n171 = property on="g_b" class="DigNum (严格)"("DisabledEnum"=w404) -> ()  [unwired: 2 in, 2 out]
            n172 = property on="Run" class="Bool"("DisabledEnum"=w409) -> ()  [unwired: 2 in, 2 out]
            n173 = property on="stop" class="Bool"("DisabledEnum"=T5."Enabled" ("禁用")) -> ()  [unwired: 2 in, 2 out]
            n174 = property on="apply" class="Bool"("DisabledEnum"=w409) -> ()  [unwired: 2 in, 2 out]
            n175 = property on="detect" class="Bool"("DisabledEnum"=w409) -> ()  [unwired: 2 in, 2 out]
            n176 = property on="detect_n" class="Bool"("DisabledEnum"=w404) -> ()  [unwired: 2 in, 2 out]
          }
          event "detect_n": Value Change {
            w425 = T5."Disabled and Grayed Out" ("禁用")
            w420 = T5."Disabled and Grayed Out" ("禁用")
            n177 = event-data() -> ()  [unwired: 1 in, 1 out]
            n178 = property class="VI"("Front Panel.Closeable"=FALSE ("前面板窗口:可关闭")) -> ()  [unwired: 2 in, 2 out]
            n179 = property on="close" class="Bool"("DisabledEnum"=w420) -> ()  [unwired: 2 in, 2 out]
            n180 = Bundle By Name(cluster=cluster{"op":string, "data":variant} {"op"="DETECT", "data"=variant}, "data"=T4 {"b"=-1.0, "e"=-1.0} ("g_data")) -> (w426:cluster{"op":string, "data":variant})
            n181 = Enqueue Element(queue=w430, element=w426) -> ()  [unwired: 2 in, 3 out]
            n182 = property on="SAM" class="Ring (严格)"("DisabledEnum"=w420) -> ()  [unwired: 2 in, 2 out]
            n183 = property on="g_e" class="DigNum (严格)"("DisabledEnum"=w420) -> ()  [unwired: 2 in, 2 out]
            n184 = property on="SJW" class="Ring (严格)"("DisabledEnum"=w420) -> ()  [unwired: 2 in, 2 out]
            n185 = property on="Run" class="Bool"("DisabledEnum"=w425) -> ()  [unwired: 2 in, 2 out]
            n186 = property on="g_b" class="DigNum (严格)"("DisabledEnum"=w420) -> ()  [unwired: 2 in, 2 out]
            n187 = property on="stop" class="Bool"("DisabledEnum"=T5."Enabled" ("禁用")) -> ()  [unwired: 2 in, 2 out]
            n188 = property on="apply" class="Bool"("DisabledEnum"=w425) -> ()  [unwired: 2 in, 2 out]
            n189 = property on="detect_n" class="Bool"("DisabledEnum"=w420) -> ()  [unwired: 2 in, 2 out]
            n190 = property on="detect" class="Bool"("DisabledEnum"=w420) -> ()  [unwired: 2 in, 2 out]
          }
          event "apply": Value Change {
            n191 = event-data() -> ()  [unwired: 1 in, 1 out]
            n192 = property on="list" class="MCListbox (严格)"() -> ("ItemSyms"=w440:i32[], "Value"=w436:i32)  [unwired: 2 in, 2 out]
            n193 = Index Array(array=w440, index=w436) -> (element=w439:i32)
            n194 = Equal?(x=w439, y=1) -> (x = y?=w437:bool)
            n195 = case shown="假" w437 {
              tunnel: w441 -> [_ w451]
              tunnel: w436 -> [_ w449]
              frame False {
                n196 = call "sub-Language-get str-const.vi"("sid"=u32 298) -> ("str"=w446:string)
                n197 = call "sub-Language-get str-const.vi"("sid"=u32 267) -> ("str"=w444:string)
                n198 = One Button Dialog(message=w446, button name ("OK")=w444) -> ()  [unwired: 1 out]
              }
              frame True {
                n199 = Bundle By Name(cluster=cluster{"op":string, "data":variant} {"op"="APPLY", "data"=variant}, "data"=w449) -> (w448:cluster{"op":string, "data":variant})
                n200 = Enqueue Element(queue=w451, element=w448) -> ()  [unwired: 2 in, 3 out]
              }
            }
          }
          event "stop": Value Change {
            n201 = event-data() -> ()  [unwired: 1 in, 1 out]
            n202 = Enqueue Element(queue=w457, element=cluster{"op":string, "data":variant} {"op"="STOP", "data"=variant}) -> ()  [unwired: 2 in, 3 out]
            n203 = property on="close" class="Bool"("DisabledEnum"=T5."Enabled" ("禁用")) -> ()  [unwired: 2 in, 2 out]
          }
          event "DevType": Value Change {
            n204 = event-data() -> ("NewVal"=w469:u32)  [unwired: 1 in]
            n205 = Equal?(x=w469, y=u32 2) -> (x = y?=w467:bool)
            n206 = Select(t=i32[] [1] ("禁用项[]"), s=w467, f=i32[] []) -> (s? t:f=w464:i32[])
            n207 = property on="Channel" class="Ring (严格)"("Disabled Items []"=w464) -> ()  [unwired: 2 in, 2 out]
          }
          event "Success": Value Change {
            w473 = T5."Disabled and Grayed Out" ("禁用")
            w474 = T5."Enabled" ("禁用")
            n208 = event-data() -> ("NewVal"=w480:bool)  [unwired: 1 in]
            n209 = control-ref of="list"() -> (w485:refnum<vi>)
            n210 = Wait (ms)(milliseconds to wait=u32 100 ("等待时间（毫秒）")) -> (millisecond timer value=w477:u32)
            n211 = Equal?(x=w484, y=1) -> (x = y?=w482:bool)
            n212 = property class="VI"("Front Panel.Closeable"=TRUE ("前面板窗口:可关闭")) -> ()  [unwired: 2 in, 2 out]
            n213 = stacked-sequence {
              tunnel: w485 -> [w491]
              tunnel: w482 -> [w490]
              tunnel: [w489] -> w481
              tunnel: w477 -> [_]
              frame #0 {
                n214 = call "BaudDetect-Make Success Info.vi"("Normal"=w490, "list"=w491) -> ("Info"=w489:string)  [unwired: 9 in]
              }
            }
            n215 = call "sub-Language-get str-const.vi"("sid"=u32 267) -> ("str"=w471:string)
            n216 = One Button Dialog(message=w481, button name ("OK")=w471) -> ()  [unwired: 1 out]
            n217 = property on="SAM" class="Ring (严格)"("DisabledEnum"=w474) -> ()  [unwired: 2 in, 2 out]
            n218 = Select(t=w474, s=w480, f=w473) -> ()  [unwired: 1 out]
            n219 = property on="SJW" class="Ring (严格)"("DisabledEnum"=w474) -> ()  [unwired: 2 in, 2 out]
            n220 = property on="close" class="Bool"("DisabledEnum"=w474) -> ()  [unwired: 2 in, 2 out]
            n221 = property on="stop" class="Bool"("DisabledEnum"=w473) -> ()  [unwired: 2 in, 2 out]
            n222 = property on="apply" class="Bool"("DisabledEnum"=w473) -> ()  [unwired: 2 in, 2 out]
            n223 = property on="detect" class="Bool"("DisabledEnum"=w474) -> ()  [unwired: 2 in, 2 out]
            n224 = property on="g_e" class="DigNum (严格)"("DisabledEnum"=w474) -> ()  [unwired: 2 in, 2 out]
            n225 = property on="g_b" class="DigNum (严格)"("DisabledEnum"=w474) -> ()  [unwired: 2 in, 2 out]
            n226 = property on="detect_n" class="Bool"("DisabledEnum"=w474) -> ()  [unwired: 2 in, 2 out]
          }
          event "help": Value Change {
            n227 = event-data() -> ()  [unwired: 1 in, 1 out]
            n228 = call "Global_Application Path.vi"() -> ("程序路径"=w497:path)  [unwired: 1 in]
            n229 = Concatenate Strings("help" ("名称或相对路径"), "\\" ("字符串"), "4.波特率侦测工具使用说明书.pdf" ("字符串")) -> (w493:string)
            n230 = Build Path(base path=w497, name or relative path=w493) -> (appended path=w496:path)
            n231 = call "Launch a File with its Default Application.vi"("File Path"=w496) -> ()  [unwired: 10 in, 1 out]
          }
        }
      }
      frame "Release" {
        n232 = case shown="真" w505 {
          frame False {
          }
          frame True {
            n233 = local read "DevType"() -> (w508:u32)
            n234 = local read "DevInd"() -> (w507:u32)
            n235 = dll-call lib="PTH1[abs ZHost_E工作Tnewcodewith eng verUSB CAN Tool2.02dataControlCAN.dll" fn="VCI_CloseDevice"("DeviceType"=w508, "DeviceInd"=w507) -> ()  [unwired: 6 in, 2 out]
          }
        }
        n236 = Enqueue Element(queue=w504, element=cluster{"op":string, "data":variant} {"op"="EXIT", "data"=variant} ("元素")) -> ()  [unwired: 2 in, 3 out]
      }
      frame "Exit" {
        n237 = control-ref of="本VI"() -> (w509:refnum<vi>)
      }
    }
  }
  n238 = Release Queue(queue=w15) -> (error out=w12:errorcluster)  [unwired: 2 in, 2 out]
  n239 = call "Exit.vi"("error in (no error)"=w12, "VI引用"=w11) -> ()  [unwired: 9 in, 1 out]
